vi "Write to Stream.vi"(8 "error in (no error)":errorcluster, 10 "Data":string, 11 "Terminal in":refnum<class "Terminal.lvclass">) -> (0 "error out":errorcluster, 3 "Terminal out":refnum<class "Terminal.lvclass">)   [LabVIEW 2020, in "Terminal.lvlib" / "Terminal.lvclass"]
uses:
  Terminal.lvclass
  Terminal.lvclass/Terminal.ctl
  <vilib>/IlluminatedG/lv-stream/Connection/Connection.lvclass
  <vilib>/IlluminatedG/lv-stream/stream/Stream.lvclass
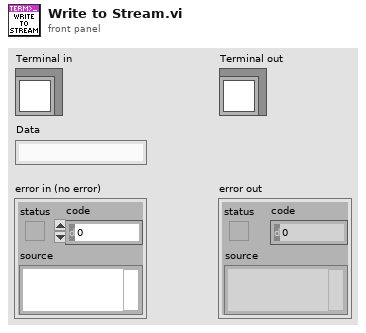
[diagram p1: front panel]
types:
  T1 = typedef "Terminal.lvlib/Terminal.lvclass/Ref Data.ctl" = cluster{"Connection":refnum<class "Connection.lvclass">, "Read Loop Running":bool, "Parse State":T2, "Terminal Options":T7, "Font Metrics":T10, "Scroll":i32, "Close Read Loop":bool, "Buffer":T11, "Pause Read Loop":bool}
  T2 = typedef "Terminal.lvlib/Terminal.lvclass/Parse State.ctl" = cluster{"Buffer State":T3, "Cursor":T4, "Attributes":T6}
  T3 = typedef "Terminal.lvlib/Terminal.lvclass/Buffer State.ctl" = cluster{"Sequence":string, "ESC":bool, "Alt Buf":bool}
  T4 = typedef "Terminal.lvlib/Terminal.lvclass/Cursor.ctl" = cluster{"Cur":T5, "Saved":T5}
  T5 = typedef "Terminal.lvlib/Terminal.lvclass/Position.ctl" = cluster{"Row":i32, "Col":i32}
  T6 = typedef "Terminal.lvlib/Text Attributes.ctl" = cluster{"FG":u32, "BG":u32, "Bold":bool, "Italic":bool, "Underline":bool, "Strike":bool, "Inverse":bool}
  T7 = typedef "Terminal.lvlib/Terminal Options.ctl" = cluster{"Implied CR with LF":bool, "Local Echo":bool, "Tab Width":i32, "Color Scheme":T8, "Default FG":T9, "Default BG":T9, "History Length":i32, "Font Face":string, "Font Size":i16, "Rows":i32, "Cols":i32}
  T8 = typedef "Terminal.lvlib/Color Scheme.ctl" = cluster{"Black":u32, "Red":u32, "Green":u32, "Yellow":u32, "Blue":u32, "Magenta":u32, "Cyan":u32, "White":u32, "Bright Black":u32, "Bright Red":u32, "Bright Green":u32, "Bright Yellow":u32, "Bright Blue":u32, "Bright Magenta":u32, "Bright Cyan":u32, "Bright White":u32}
  T9 = typedef "Terminal.lvlib/Color.ctl" = i8
  T10 = typedef "Terminal.lvlib/Terminal.lvclass/Font Metrics.ctl" = cluster{"Width":i16, "Height":i16}
  T11 = typedef "Terminal.lvlib/Buffer.ctl" = enum16{"Primary", "Alternate"}
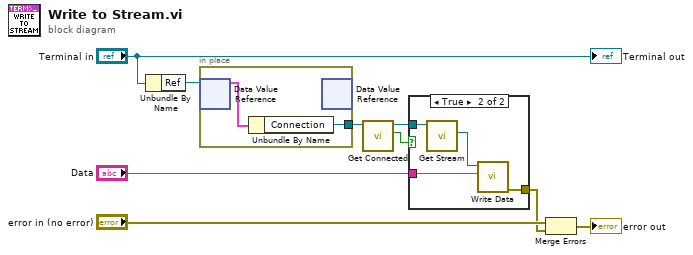
[diagram p0: block diagram]
diagram:
  n1 = Unbundle By Name("Terminal in") -> ("Ref"=w8:refnum<data-value>)
  n2 = in-place {
    in-place-border: [w10] -> w7
    n3 = in-place-dvr #1(w8) -> (w11:T1)  [unwired: 1 out]
    n4 = Unbundle By Name(w11) -> ("Connection"=w10:refnum<class "Connection.lvclass">)
    n5 = in-place-dvr #1() -> ()  [unwired: 1 in, 2 out]
  }
  n6 = call <vilib>:"Get Connected.vi"("Connection in"=w7) -> ("Connected"=w5:bool, "Connection out"=w6:refnum<class "Connection.lvclass">)  [unwired: 8 in, 1 out]
  n7 = case shown="True" w5 {
    tunnel: [_ w14] -> w1
    tunnel: w6 -> [_ w13]
    tunnel: "Data" -> [_ w12]
    frame False {
    }
    frame True {
      n8 = call-dynamic "Get Stream.vi"("Connection in"=w13) -> ("Stream"=w15:refnum<class "Stream.lvclass">)  [unwired: 8 in, 2 out]
      n9 = call <vilib>:"Write Data.vi"("Data"=w12, "Stream in"=w15) -> ("error out"=w14:errorcluster)  [unwired: 8 in, 1 out]
    }
  }
  n10 = Merge Errors("error in (no error)", w1) -> (→"error out":errorcluster)
  "Terminal out" <- "Terminal in"
